vi "DefColors Write.vi"(4 "error in (no error)":errorcluster, 5 "Value":u32[](array[numeric]), 6 "Container State":T6, 7 "Display State In":T1) -> (0 "error out":errorcluster, 3 "Display State Out":T1)   [LabVIEW 2020, in "KTable.xctl"]
uses:
  KTable.xctl
  <vilib>/_xctls/Container State.ctl
  State.ctl
  ColumnSpec.ctl
  ColumnType.ctl
  Table Properties.ctl
  Events.ctl
  Event Data.ctl
  Event Type.ctl
  Array Manipulation VIs/Array-Dimensions (2D string).vi
  <vilib>/_xctls/XControlSupport.lvlib
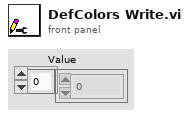
[diagram p1: front panel]
types:
  T1 = typedef "KTable.xctl/State.ctl" = cluster{"Columns":T2[], "Listbox":refnum<vi>, "Default row":string[], "Properties":T4, "Events":T5, "Locked":bool[][], "Size":cluster{"Rows":i32, "Columns":i32}, "rings":i32[][], "DefColors":u32[]}
  T2 = typedef "KTable.xctl/ColumnSpec.ctl" = cluster{"Name":string, "Type":T3, "Width":i32, "Strings":string[], "Position":enum16{"Left", "Center", "Right"}, "locked":bool, "cds":cluster{"Strings":string[]}[][], "Hide NaN":bool}
  T3 = typedef "KTable.xctl/ColumnType.ctl" = enum16{"String", "Enum", "Int", "Double", "Boolean", "Ring", "Formula", "Color"}
  T4 = typedef "KTable.xctl/Table Properties.ctl" = cluster{"Vertical scrollbar":bool, "User add/delete":bool, "Max rows":i32, "Row headers":bool}
  T5 = typedef "KTable.xctl/Events.ctl" = cluster{"Items Changed":refnum<user-event>}
  T6 = typedef "XControlSupport.lvlib/Container State.ctl" = cluster{"Indicator?":bool, "Run Mode?":bool, " Refnum":refnum<vi>}
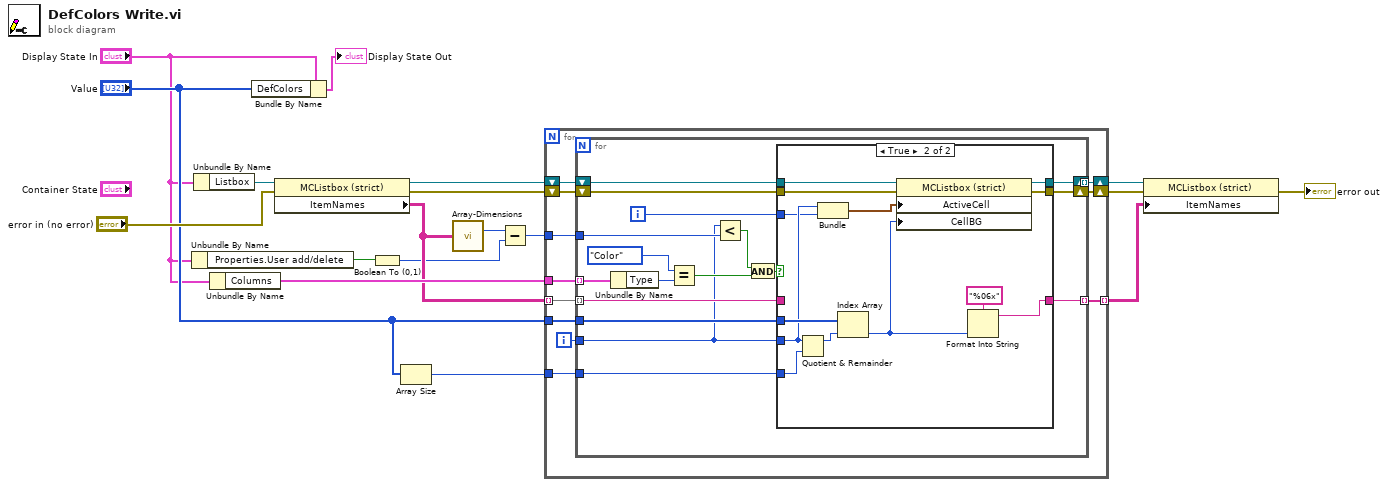
[diagram p0: block diagram]
diagram:
  n1 = Unbundle By Name("Display State In") -> ("Properties.User add/delete"=w4:bool)
  n2 = Unbundle By Name("Display State In") -> ("Listbox"=w17:refnum<vi>)
  n3 = Unbundle By Name("Display State In") -> ("Columns"=w15:T2[])
  n4 = Bundle By Name(cluster="Display State In", "DefColors"="Value") -> (→"Display State Out":T1)
  n5 = property class="MCListbox (strict)"(reference=w17, error in="error in (no error)") -> (reference out=w10:refnum<vi>, error out=w7:errorcluster, "ItemNames"=w6:string[][])
  n6 = Boolean To (0,1)(Boolean=w4) -> (0, 1=w2:i16)
  n7 = Array Size(array="Value") -> (size(s)=w13:i32)
  n8 = call-poly "Array-Dimensions.vi"("2D Array"=w6) -> ("# rows"=w3:i32)  [unwired: 13 in, 1 out]
  n9 = Subtract(x=w3, y=w2) -> (x-y=w1:i32)
  n10 = for {
    tunnel: w6 -> [w29] mode=indexing
    tunnel: w15 -> [w28]
    tunnel: "Value" -> [w26]
    tunnel: w13 -> [w25]
    tunnel: [w24] -> w11 mode=indexing
    shift-right: [w22] -> w9
    shift-left: w10 -> [w23]
    shift-right: [w21] -> w8
    shift-left: w7 -> [w20]
    tunnel: w1 -> [w19]
    i -> [w27]
    n11 = for {
      tunnel: w29 -> [w45] mode=indexing
      tunnel: w28 -> [w46] mode=indexing
      tunnel: w27 -> [w30]
      tunnel: w26 -> [w44]
      tunnel: w25 -> [w43]
      tunnel: [w42] -> w24 mode=indexing
      shift-right: [w40] -> w22
      shift-left: w23 -> [w41]
      tunnel: [w40] -> _ mode=indexing
      shift-right: [w39] -> w21
      shift-left: w20 -> [w38]
      tunnel: w19 -> [w33]
      i -> [w34]
      n12 = Unbundle By Name(w46) -> ("Type"=w37:T3)
      n13 = Equal?(x=ColumnType."Color", y=w37) -> (x = y?=w35:bool)
      n14 = Less?(x=w30, y=w33) -> (x < y?=w32:bool)
      n15 = And(x=w32, y=w35) -> (x .and. y?=w31:bool)
      n16 = case shown="True" w31 {
        tunnel: w45 -> [w49 _]
        tunnel: w30 -> [_ w53]
        tunnel: w44 -> [_ w60]
        tunnel: w43 -> [_ w62]
        tunnel: [w49 w58] -> w42
        tunnel: w41 -> [w48 w57]
        tunnel: [w48 w55] -> w40
        tunnel: [w47 w54] -> w39
        tunnel: w38 -> [w47 w56]
        tunnel: w34 -> [_ w52]
        frame False {
        }
        frame True {
          n17 = Quotient & Remainder(x=w53, y=w62) -> (x-y*floor(x/y)=w61:i32)  [unwired: 1 out]
          n18 = Bundle(w53, w52) -> (w51:cluster{i32, i32})  [unwired: 1 in]
          n19 = Index Array(array=w60, index=w61) -> (element=w50:u32)
          n20 = property class="MCListbox (strict)"(reference=w57, error in=w56, "ActiveCell"=w51, "CellBG"=w50) -> (reference out=w55:refnum<vi>, error out=w54:errorcluster)
          n21 = Format Into String(format string="%06x", w50) -> (resulting string=w58:string)  [unwired: 2 in, 1 out]
        }
      }
    }
  }
  n22 = property class="MCListbox (strict)"(reference=w9, error in=w8, "ItemNames"=w11) -> (error out=→"error out":errorcluster)  [unwired: 1 out]
